vi "FP_VIG_Controls and Names.vi"(8 "Error":errorcluster, 11 "MAin Ref\nFirst Time only":refnum<vi>) -> (0 "Error Out":errorcluster, 2 "FP Names Out":string[](array[string]), 3 "FP Controls Out":refnum<vi>[](array[refnum]), 5 "FrontPanel Out":refnum<vi>)   [LabVIEW 2020]
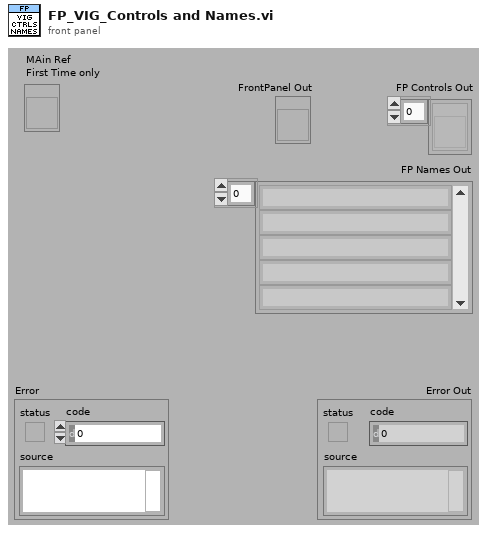
[diagram p1: front panel]
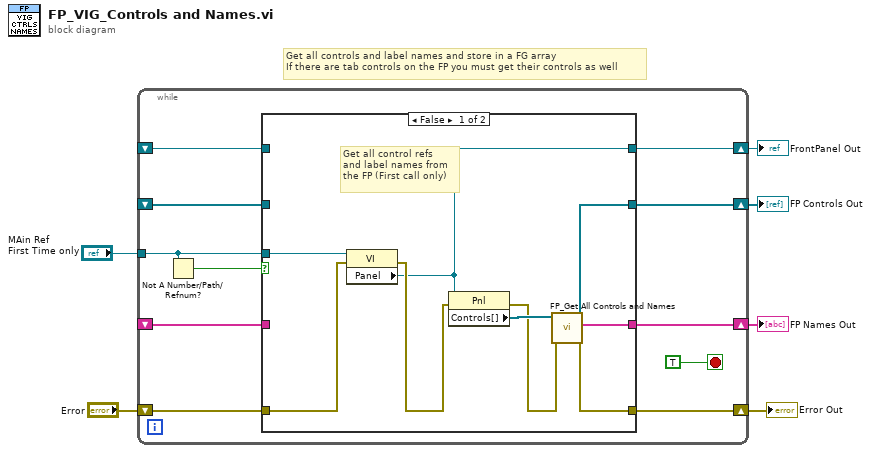
[diagram p0: block diagram]
diagram:
  # "Get all controls and label names and store in a FG array\nIf there are tab controls on the FP you must get their controls as well"
  n1 = while {
    shift-right: [w17] -> w6
    shift-left: _ -> [w8]
    shift-right: [w16] -> w5
    shift-left: _ -> [w15]
    shift-right: [w12] -> w3
    shift-left: "Error" -> [w13]
    shift-right: [w11] -> w2
    shift-left: _ -> [w10]
    tunnel: "MAin Ref\nFirst Time only" -> [w9]
    stop <- TRUE stop-if-true
    n2 = Not A Number/Path/Refnum?(number/path/refnum=w9) -> (NaN/Path/Refnum?=w7:bool)
    n3 = case shown="False" w7 {
      tunnel: [w25 w30] -> w17
      tunnel: [w24 w29] -> w16
      tunnel: w15 -> [_ w29]
      tunnel: w8 -> [_ w30]
      tunnel: w13 -> [w21 w28]
      tunnel: [w23 w28] -> w12
      tunnel: [w19 w27] -> w11
      tunnel: w10 -> [_ w27]
      tunnel: w9 -> [w18 _]
      frame False {
        # "Get all control refs\nand label names from\nthe FP (First call only)"
        n4 = property class="VI"(reference=w18, error in=w21) -> (error out=w20:errorcluster, "Panel"=w19:refnum<vi>)  [unwired: 1 out]
        n5 = property class="Pnl"(reference=w19, error in=w20) -> (error out=w22:errorcluster, "Controls[]"=w26:refnum<vi>[])  [unwired: 1 out]
        n6 = call "FP_Get All Controls and Names.vi"("Error"=w22, "Generics"=w26) -> ("Error Out"=w23:errorcluster, "Names Out"=w24:string[], "Controls[] Out"=w25:refnum<vi>[])  [unwired: 7 in]
      }
      frame True {
      }
    }
  }
  "FP Controls Out" <- w6
  "FP Names Out" <- w5
  "Error Out" <- w3
  "FrontPanel Out" <- w2
